vi "_littletool_EEPROM_vna_wmg.vi"(1 "read buffer":string, 2 "inputArray":u8[](array[numeric]) format="%.0x") -> (0 "数组":string[][](array[string]))   [LabVIEW 2011]
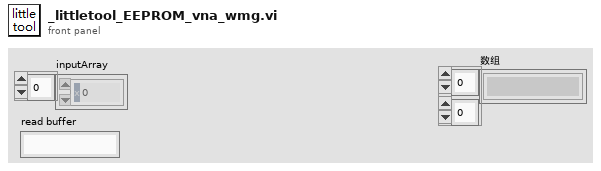
[diagram p1: front panel]
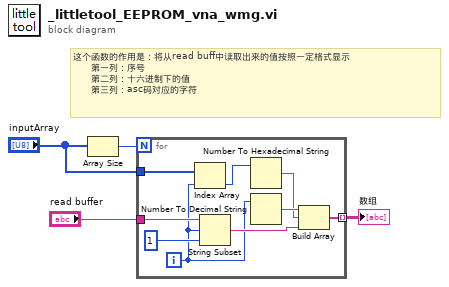
[diagram p0: block diagram]
diagram:
  # "这个函数的作用是：将从read buff中读取出来的值按照一定格式显示\n      第一列：序号\n      第二列：十六进制下的值\n      第三列：asc码对应的字符"
  n1 = Array Size(array="inputArray") -> (size(s)=w4:i32)
  n2 = for {
    N: w4 -> [_]
    tunnel: "inputArray" -> [w13]
    tunnel: "read buffer" -> [w12]
    tunnel: [w5] -> w1 mode=indexing
    i -> [w8]
    n3 = Index Array(array=w13, index=w8) -> (element=w9:u8)
    n4 = String Subset(string=w12, offset (0)=w8, length (rest)=1 ("length (rest)")) -> (substring=w10:string)
    n5 = Number To Hexadecimal String(2:w9) -> (0:w6:string)  [unwired: 1 in]
    n6 = Number To Decimal String(number=w8) -> (decimal integer string=w7:string)  [unwired: 1 in]
    n7 = Build Array(w7, w6, w10) -> (w5:string[])
  }
  "数组" <- w1
